vi "draw xy graph Ellipse.vi"(6 "ellipse description":T1={"X axis radius (b4 rot)"=57.41811175337187, "Y Axis radius (b4 rot"=31.984585741811177, "x-Shift"=-21.098265895953755, "y-shift"=0.48169556840077216, "rotation"=59.653179190751445} {"rotation" scale=0.0..180.0; "y-shift" scale=-50.0..50.0; "x-Shift" scale=-50.0..50.0; "Y Axis radius (b4 rot" scale=0.0..100.0; "X axis radius (b4 rot)" scale=0.0..100.0}) -> (1 "Elipse points":cluster{i32, i32}[](array[cluster]), 2 "XY Graph 2":cluster{dbl[], dbl[]}(graph))   [LabVIEW 2013]
uses:
  ellipse description.ctl
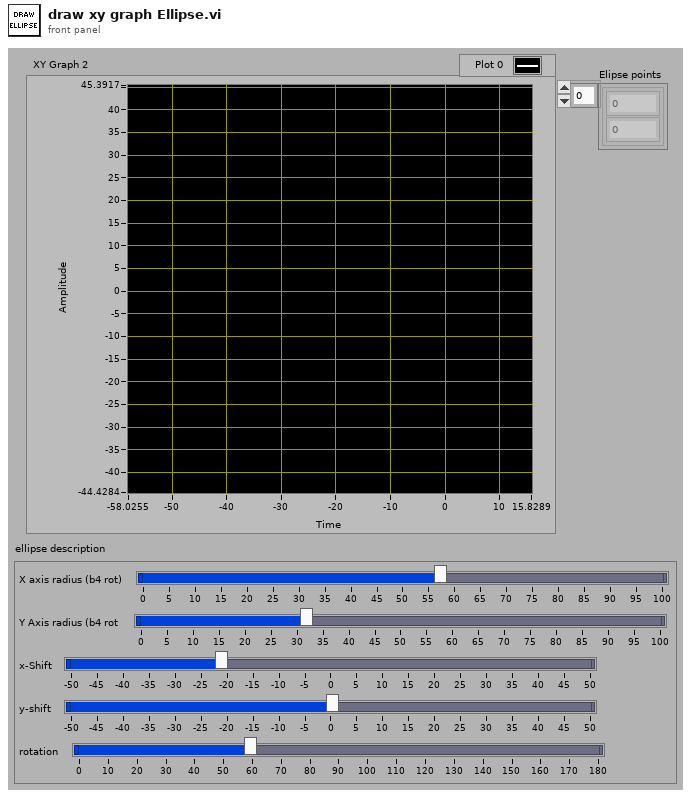
[diagram p1: front panel]
types:
  T1 = typedef "ellipse description.ctl" = cluster{"X axis radius (b4 rot)":dbl, "Y Axis radius (b4 rot":dbl, "x-Shift":dbl, "y-shift":dbl, "rotation":dbl}
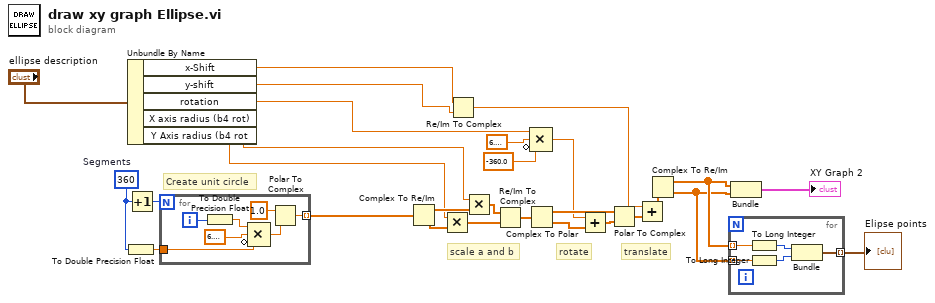
[diagram p0: block diagram]
diagram:
  w27 = 360  # Segments
  # "translate"
  # "rotate"
  # "scale a and b"
  # "Create unit circle"
  n1 = To Double Precision Float(number=w27) -> (double precision float=w26:dbl)
  n2 = Increment(x=w27) -> (x+1=w28:i32)
  n3 = Unbundle By Name("ellipse description") -> ("x-Shift"=w6:dbl, "y-shift"=w5:dbl, "rotation"=w4:dbl, "X axis radius (b4 rot)"=w23:dbl, "Y Axis radius (b4 rot"=w7:dbl)
  n4 = for {
    N: w28 -> [_]
    tunnel: w26 -> [w29]
    tunnel: [w33] -> w25 mode=indexing
    i -> [w34]
    n5 = To Double Precision Float(number=w34) -> (double precision float=w31:dbl)
    n6 = Compound Arithmetic op=MULTIPLY(w31, 6.283185307179586, invert w29) -> (w30:dbl)
    n7 = Polar To Complex(1:w30, 2:1.0 ("r")) -> (0:w33:cdb)
  }
  n8 = Complex To Re/Im(x + iy=w25) -> (x=w21:dbl[], y=w22:dbl[])
  n9 = Multiply(x=w7, y=w22) -> (x*y=w19:dbl[])
  n10 = Re/Im To Complex(1:w5, 2:w6) -> (0:w12:cdb)
  n11 = Multiply(x=w23, y=w21) -> (x*y=w20:dbl[])
  n12 = Re/Im To Complex(1:w19, 2:w20) -> (0:w18:cdb[])
  n13 = Complex To Polar(r * e^(i*theta)=w18) -> (r=w16:dbl[], theta=w17:dbl[])
  n14 = Compound Arithmetic op=MULTIPLY(w4, 6.283185307179586, invert -360.0 ("y")) -> (w9:dbl)
  n15 = Add(x=w9, y=w17) -> (x+y=w15:dbl[])
  n16 = Polar To Complex(1:w15, 2:w16) -> (0:w14:cdb[])
  n17 = Add(x=w12, y=w14) -> (x+y=w13:cdb[])
  n18 = Complex To Re/Im(x + iy=w13) -> (x=w3:dbl[], y=w2:dbl[])
  n19 = for {
    tunnel: w3 -> [w39] mode=indexing
    tunnel: w2 -> [w36] mode=indexing
    tunnel: [w40] -> w1 mode=indexing
    n20 = To Long Integer(number=w39) -> (32bit integer=w38:i32)
    n21 = To Long Integer(number=w36) -> (32bit integer=w37:i32)
    n22 = Bundle(w38, w37) -> (w40:cluster{i32, i32})  [unwired: 1 in]
  }
  "Elipse points" <- w1
  n23 = Bundle(w3, w2) -> (→"XY Graph 2":cluster{dbl[], dbl[]})  [unwired: 1 in]
